vi "To-string.vi"(8 "error in (no error)":errorcluster, 11 "Sequence in":refnum<class "Action-sequence.lvclass">) -> (0 "error out":errorcluster, 2 "Action string array":string[][](array[string]), 3 "Sequence out":refnum<class "Action-sequence.lvclass">)   [LabVIEW 2013, in "PowderDeposition.lvlib" / "Action-sequence.lvclass"]
uses:
  Action-sequence.lvclass
  Action-sequence.lvclass/Action-sequence.ctl
  Action/Action.lvclass
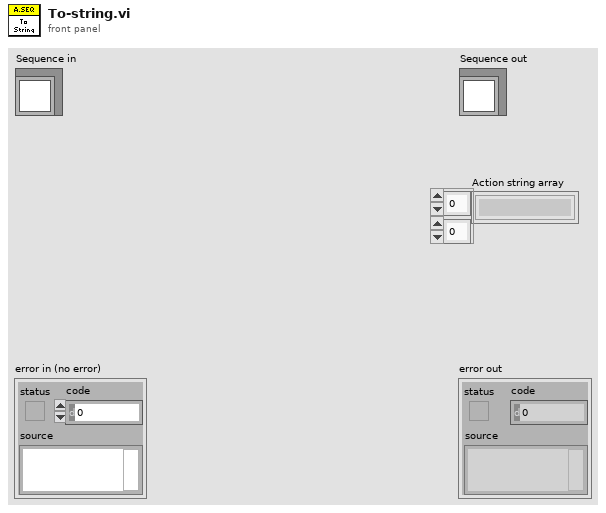
[diagram p1: front panel]
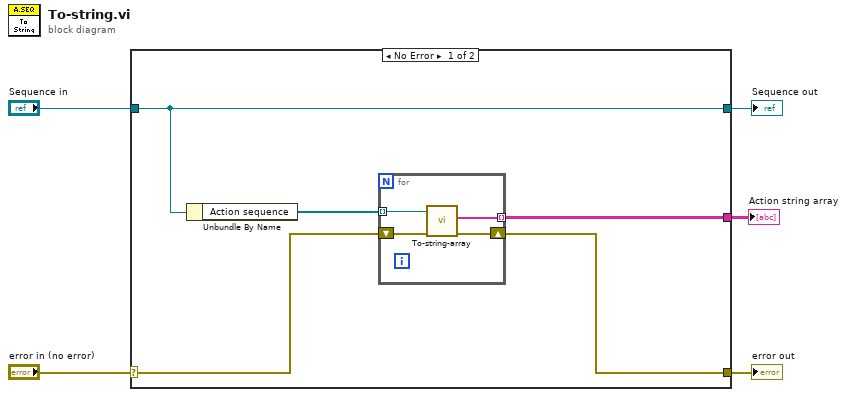
[diagram p0: block diagram]
diagram:
  n1 = case shown="No Error" "error in (no error)" {
    selector: "error in (no error)" -> [w7 w16]
    tunnel: [w6 w16] -> w4
    tunnel: [w10 w15] -> w2
    tunnel: "Sequence in" -> [w10 w15]
    tunnel: [w8 _] -> w1
    frame No Error {
      n2 = Unbundle By Name(w10) -> ("Action sequence"=w9:refnum<class "Action.lvclass">[])
      n3 = for {
        tunnel: w9 -> [w14] mode=indexing
        shift-right: [w12] -> w6
        shift-left: w7 -> [w13]
        tunnel: [w11] -> w8 mode=indexing
        n4 = call-dynamic "To-string-array.vi"("error in (no error)"=w13, "Action in"=w14) -> ("error out"=w12:errorcluster, "Action string array"=w11:string[])  [unwired: 7 in, 1 out]
      }
    }
    frame Error {
    }
  }
  "error out" <- w4
  "Sequence out" <- w2
  "Action string array" <- w1
